vi "ImageButtonWriteProp.vi"(4 "error in (no error)":errorcluster, 5 "Value":i32(ring)=13 items=["Left", "LeftBig", "LeftSmall", "Right", "RightBig", "RightSmall", "Up", "UpBig", "UpSmall", "Down", "DownBig", "DownSmall", "Zero", "Play", "Pause", "Load", "Lower", "Raise", "Home", "Home2"], 6 "Container State":T2, 7 "Display State In":T1={"image"=13} {"image" items=["Left", "LeftBig", "LeftSmall", "Right", "RightBig", "RightSmall", "Up", "UpBig", "UpSmall", "Down", "DownBig", "DownSmall", "Zero", "Play", "Pause", "Load", "Lower", "Raise", "Home", "Home2"]}) -> (0 "error out":errorcluster, 3 "Display State Out":T1={"image"=13} {"image" items=["Left", "LeftBig", "LeftSmall", "Right", "RightBig", "RightSmall", "Up", "UpBig", "UpSmall", "Down", "DownBig", "DownSmall", "Zero", "Play", "Pause", "Load", "Lower", "Raise", "Home", "Home2"]})   [LabVIEW 2020, in "ImageButton2.xctl"]
uses:
  <vilib>/_xctls/Container State.ctl
  ImageButton2.xctl
  <vilib>/_xctls/XControlSupport.lvlib
  ImageButtonState.ctl
panel:
  # "Replace the Value Control below with a Control of desired type.\nDo not remove this Control or the others from the connector pane.\nDo not change the connector pane pattern.\nThe Value control should always be the third terminal from top on the input side in the connector pane."
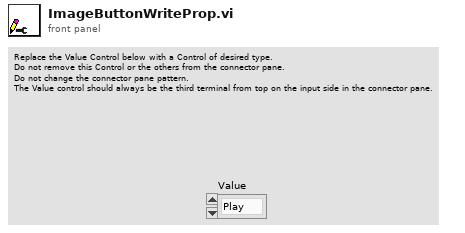
[diagram p1: front panel]
types:
  T1 = typedef "ImageButton2.xctl/ImageButtonState.ctl" = cluster{"image":i32}
  T2 = typedef "XControlSupport.lvlib/Container State.ctl" = cluster{"Indicator?":bool, "Run Mode?":bool, " Refnum":refnum<vi>}
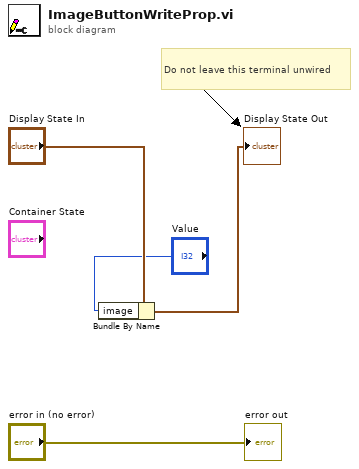
[diagram p0: block diagram]
diagram:
  # "Do not leave this terminal unwired"
  n1 = Bundle By Name(cluster="Display State In", "image"="Value") -> (→"Display State Out":T1)
  "error out" <- "error in (no error)"
